vi "GetFRSignalAndChDataRef.vi"(7 "Access":T3, 8 "error in (no error)":errorcluster, 10 "Channel Refs":T2[](array[typedef]) format="%.0x", 11 "Device Ref in":T2 format="%.0x") -> (0 "error out":errorcluster, 1 "FR Signals":refnum<k21>[](array[refnum]), 2 "Channel Data Ref":T1[](array[typedef]) format="%.0x", 3 "Device Ref out":T2 format="%.0x")   [LabVIEW 2020, in "FlexRay Custom Device Engine.lvlib"]
uses:
  FlexRay Custom Device Engine.lvlib
  <vilib>/NI VeriStand/Custom Device API/Data Access Type.ctl
  <vilib>/NI VeriStand/Custom Device API/Custom Device Item Ref.ctl
  <vilib>/NI VeriStand/Custom Device API/Data Reference.ctl
  Shared/Constants.vi
  <vilib>/NI VeriStand/Custom Device API/Get Item Property (Variant).vi
  <vilib>/NI VeriStand/Custom Device API/Custom Device API.lvlib
  Shared/FlexRay Custom Device Shared.lvlib
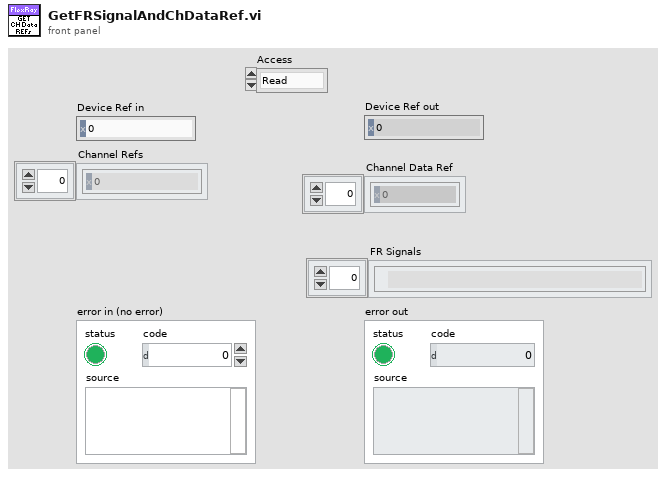
[diagram p1: front panel]
types:
  T1 = typedef "Custom Device API.lvlib/Data Reference.ctl" = i32
  T2 = typedef "Custom Device API.lvlib/Custom Device Item Ref.ctl" = u64
  T3 = typedef "Custom Device API.lvlib/Data Access Type.ctl" = enum16{"Read", "Write"}
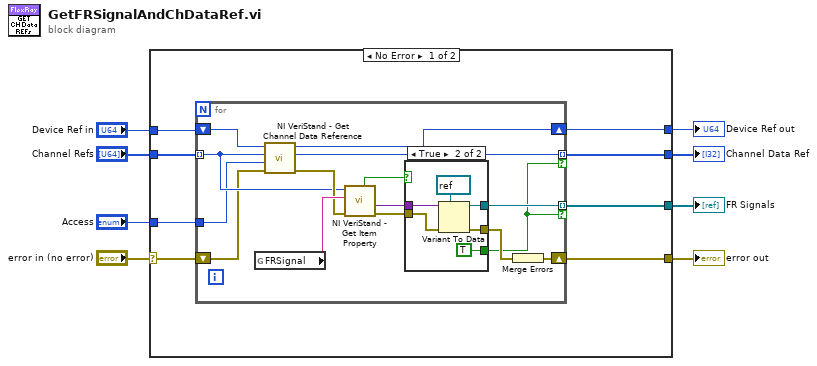
[diagram p0: block diagram]
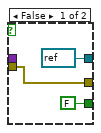
[diagram p2: hidden frame]
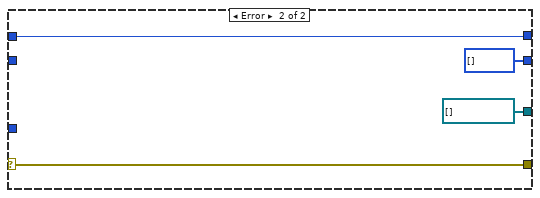
[diagram p3: hidden frame]
diagram:
  n1 = case shown="No Error" "error in (no error)" {
    selector: "error in (no error)" -> [w9 w44]
    tunnel: "Access" -> [w16 _]
    tunnel: [w15 w44] -> w7
    tunnel: [w14 w43] -> w6
    tunnel: "Device Ref in" -> [w13 w43]
    tunnel: "Channel Refs" -> [w12 _]
    tunnel: [w11 T1[] []] -> w3
    tunnel: [w10 refnum<k21>[] []] -> w2
    frame No Error {
      n2 = for {
        shift-right: [w24] -> w14
        shift-left: w13 -> [w31]
        tunnel: w12 -> [w21] mode=indexing
        shift-right: [w25] -> w15
        shift-left: w9 -> [w19]
        tunnel: [w20] -> w11 mode=indexing if=w18
        tunnel: [w26] -> w10 mode=indexing if=w18
        tunnel: w16 -> [w17]
        n3 = global read "Constants.vi" "FRSignal"() -> (w30:string)
        n4 = call <vilib>:"NI VeriStand - Get Channel Data Reference.vi"("error in (no error)"=w19, "Access"=w17, "Channel Ref in"=w21, "Device Ref in"=w31) -> ("error out"=w23:errorcluster, "Channel Data Reference"=w20:T1, "Device Ref out"=w24:T2)  [unwired: 5 out]
        n5 = call-poly <vilib>:"NI VeriStand - Get Item Property.vi"("error in (no error)"=w23, "Property Name"=w30, "Item Ref in"=w21) -> ("error out"=w28:errorcluster, "Value"=w29:variant, "Found?"=w22:bool)  [unwired: 5 in, 1 out]
        n6 = case shown="True" w22 {
          tunnel: w29 -> [_ w40]
          tunnel: w28 -> [w34 w38]
          tunnel: [w34 w37] -> w27
          tunnel: [refnum<k21> refnum ("XNET Signal") w36] -> w26
          tunnel: [FALSE TRUE] -> w18
          frame False {
          }
          frame True {
            n7 = Variant To Data(error in=w38, type=refnum<k21> refnum ("XNET Signal"), Variant=w40) -> (data=w36:refnum<k21>, error out=w37:errorcluster)
          }
        }
        n8 = Merge Errors(w27) -> (w25:errorcluster)
      }
    }
    frame Error {
    }
  }
  "error out" <- w7
  "Device Ref out" <- w6
  "Channel Data Ref" <- w3
  "FR Signals" <- w2
